vi "Magnet Shutdown.vi"   [LabVIEW 2010]
uses:
  <instrlib>/Keithley 2400/Keithley 24XX.lvlib
types:
  T1 = typedef "niSE SessionRefnum.ctl" = refnum<k1>
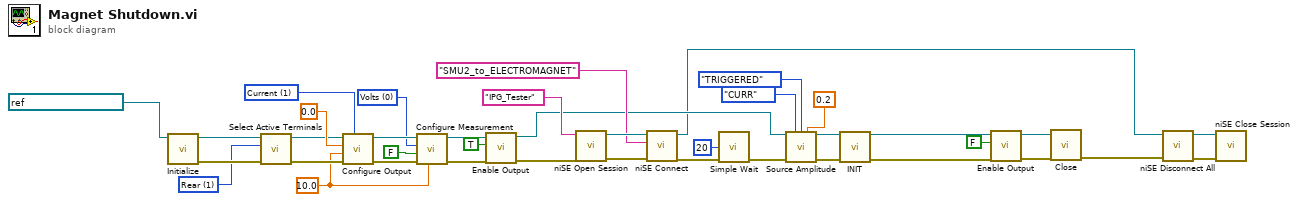
[diagram p0: block diagram]
diagram:
  w1 = u16 1 items=["Voltage", "Current"] ("Source Mode  (0: Voltage)")
  w30 = u16 0 items=["Volts", "Current", "Resistance"] ("Function (0: Volts)")
  w33 = u16 1 items=["Front", "Rear"] ("Active Terminals (0: Front)")
  w25 = 10.0 ("Compliance  Level (0.1)")
  n1 = call <instrlib>:"Initialize.vi"("VISA resource name"=refnum<visa-resource-name> "GPIB0::10::INSTR") -> ("error out"=w35:errorcluster, "VISA resource name out"=w37:refnum<visa-resource-name>)  [unwired: 9 in]
  n2 = call <instrlib>:"Select Active Terminals.vi"("error in (no error)"=w35, "Active Terminals (0: Front)"=w33, "VISA resource name"=w37) -> ("error out"=w34:errorcluster, "VISA resource name out"=w36:refnum<visa-resource-name>)  [unwired: 7 in]
  n3 = call <instrlib>:"Configure Output.vi"("Source Mode  (0: Voltage)"=w1, "error in (no error)"=w34, "Compliance  Level (0.1)"=w25, "Output Level (0)"=0.0, "VISA resource name"=w36) -> ("error out"=w31:errorcluster, "VISA resource name out"=w32:refnum<visa-resource-name>)  [unwired: 5 in]
  n4 = call <instrlib>:"Configure Measurement.vi"("Manual Range (1.0)"=w25, "error in (no error)"=w31, "Enable Auto Range (T:Enable)"=FALSE, "Function (0: Volts)"=w30, "VISA resource name"=w32) -> ("error out"=w27:errorcluster, "VISA resource name out"=w28:refnum<visa-resource-name>)  [unwired: 5 in]
  n5 = call <instrlib>:"Enable Output.vi"("error in (no error)"=w27, "Enable Output (T: Enable)"=TRUE, "VISA resource name"=w28) -> ("error out"=w16:errorcluster, "VISA resource name out"=w13:refnum<visa-resource-name>)  [unwired: 7 in]
  n6 = call <vilib>:"niSE Open Session.vi"("error in (no error)"=w16, "Virtual Device Name (SwitchConfiguration1)"="IPG_Tester") -> ("error out"=w15:errorcluster, "NISE Session (out)"=w24:T1)  [unwired: 4 in]
  n7 = call <vilib>:"niSE Connect.vi"("error in (no error)"=w15, "Connection Specification (\"\")"="SMU2_to_ELECTROMAGNET" ("Connection Specification (\"\")"), "NISE Session (in)"=w24) -> ("error out"=w14:errorcluster, "NISE Session (out)"=w5:T1)  [unwired: 7 in]
  n8 = call "Simple Wait.vi"("mS"=u32 20, "error in"=w14) -> ("error out"=w17:errorcluster)  [unwired: 12 in, 1 out]
  n9 = call "Source Amplitude.vi"("VISA resource name"=w13, "Source Function"=enum16{"CURR", "VOLT"}."CURR", "Mode"=enum16{"IMM", "TRIGGERED"}."TRIGGERED", "Source Level"=0.2, "error in (no error)"=w17) -> ("VISA resource name out"=w20:refnum<visa-resource-name>, "error out"=w19:errorcluster)  [unwired: 9 in]
  n10 = call "INIT.vi"("VISA resource name"=w20, "error in (no error)"=w19) -> ("VISA resource name out"=w4:refnum<visa-resource-name>, "error out"=w3:errorcluster)  [unwired: 12 in]
  n11 = call <instrlib>:"Enable Output.vi"("error in (no error)"=w3, "Enable Output (T: Enable)"=FALSE, "VISA resource name"=w4) -> ("error out"=w7:errorcluster, "VISA resource name out"=w6:refnum<visa-resource-name>)  [unwired: 7 in]
  n12 = call <instrlib>:"Close.vi"("error in (no error)"=w7, "VISA resource name"=w6) -> ("error out"=w2:errorcluster)  [unwired: 9 in]
  n13 = call <vilib>:"niSE Disconnect All.vi"("error in (no error)"=w2, "NISE Session (in)"=w5) -> ("error out"=w10:errorcluster, "NISE Session (out)"=w9:T1)  [unwired: 4 in]
  n14 = call <vilib>:"niSE Close Session.vi"("error in (no error)"=w10, "NISE Session (in)"=w9) -> ()  [unwired: 5 in, 1 out]
